vi "delete z slices tabs.vi"(8 "error in":errorcluster, 10 "Crop Z":cluster{"sl1":i32, "sl2":i32}={"sl1"=0, "sl2"=3}, 11 "File Table Folder":path) -> (0 "error out":errorcluster)   [LabVIEW 2023]
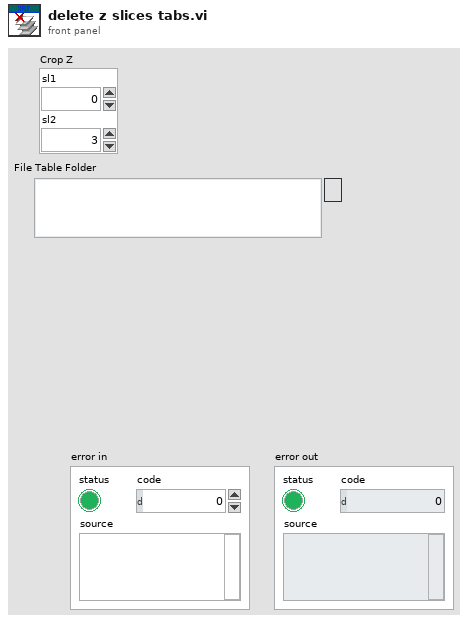
[diagram p1: front panel]
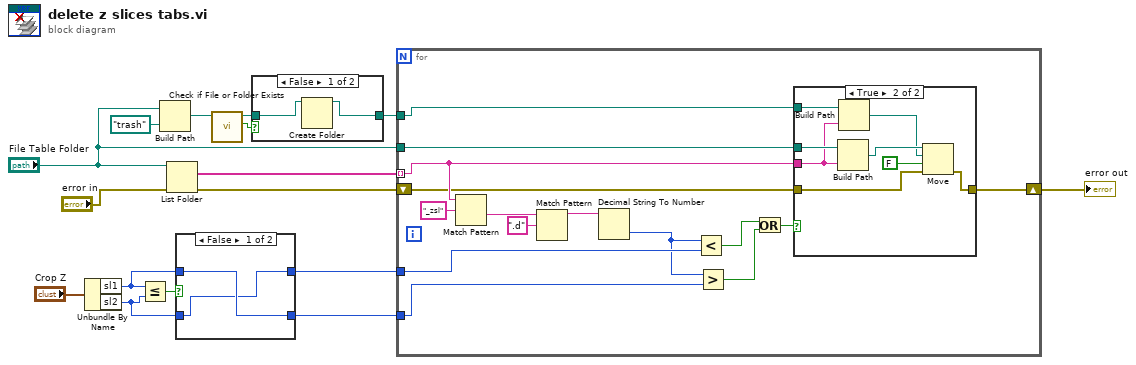
[diagram p0: block diagram]
diagram:
  n1 = Unbundle By Name("Crop Z") -> ("sl1"=w10:i32, "sl2"=w8:i32)
  n2 = Less Or Equal?(x=w10, y=w8) -> (x <= y?=w11:bool)
  n3 = Build Path(base path="File Table Folder", name or relative path=path "trash") -> (appended path=w4:path)
  n4 = List Folder(path="File Table Folder", error in="error in") -> (filenames=w15:string[], error out=w13:errorcluster)  [unwired: 2 in, 2 out]
  n5 = case shown="False" w11 {
    tunnel: [w17 w20] -> w9
    tunnel: w10 -> [w18 w20]
    tunnel: [w18 w19] -> w7
    tunnel: w8 -> [w17 w19]
    frame False {
    }
    frame True {
    }
  }
  n6 = call <vilib>:"Check if File or Folder Exists.vi"("path"=w4) -> ("file or folder exists?"=w3:bool, "dup path"=w2:path)  [unwired: 8 in, 1 out]
  n7 = case shown="False" w3 {
    tunnel: [w21 w23] -> w1
    tunnel: w2 -> [w22 w23]
    frame False {
      n8 = Create Folder(path (use dialog)=w22) -> (created path=w21:path)  [unwired: 2 in, 2 out]
    }
    frame True {
    }
  }
  n9 = for {
    tunnel: w15 -> [w35] mode=indexing
    shift-right: [w32] -> w12
    shift-left: w13 -> [w34]
    tunnel: w9 -> [w38]
    tunnel: w7 -> [w37]
    tunnel: "File Table Folder" -> [w36]
    tunnel: w1 -> [w33]
    n10 = Match Pattern(string=w35, regular expression="_zsl") -> (after substring=w29:string)  [unwired: 1 in, 3 out]
    n11 = Match Pattern(string=w29, regular expression=".d") -> (before substring=w27:string)  [unwired: 1 in, 3 out]
    n12 = Decimal String To Number(string=w27) -> (number=w24:i32)  [unwired: 2 in, 1 out]
    n13 = Less?(x=w24, y=w38) -> (x < y?=w26:bool)
    n14 = Greater?(x=w24, y=w37) -> (0:w25:bool)
    n15 = Or(x=w26, y=w25) -> (x .or. y?=w28:bool)
    n16 = case shown="True" w28 {
      tunnel: w36 -> [_ w47]
      tunnel: w34 -> [w39 w45]
      tunnel: w33 -> [_ w43]
      tunnel: w35 -> [_ w42]
      tunnel: [w39 w40] -> w32
      frame False {
      }
      frame True {
        n17 = Build Path(base path=w47, name or relative path=w42) -> (appended path=w44:path)
        n18 = Build Path(base path=w43, name or relative path=w42) -> (appended path=w41:path)
        n19 = Move(source path=w44, error in=w45, 9:FALSE ("overwrite (F)"), 10:w41) -> (error out=w40:errorcluster)  [unwired: 1 in, 2 out]
      }
    }
  }
  "error out" <- w12
